vi "Tx Disable channel logic 1ch.vi"(6 "ready for output":bool, 9 "input valid":bool, 10 "data in":u32[](array[numeric])=[0, 0, 0, 0]) -> (0 "enable new data":bool, 1 "output valid":bool, 2 "data out":u32[](array[numeric]))   [LabVIEW 2025, in "niUSRP Stream Control (DMA) v1 FPGA.lvclass"]
uses:
  niUSRP Stream Control (DMA) v1 FPGA.lvclass
  niUSRP Stream Control (DMA) v1 FPGA.lvclass/niUSRP Stream Control (DMA) v1 FPGA.ctl
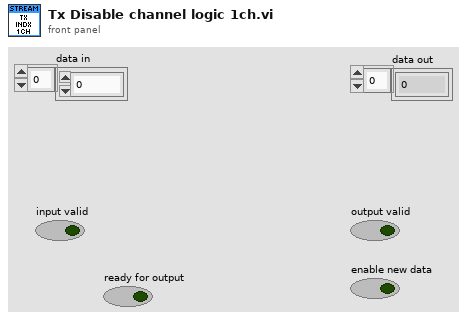
[diagram p1: front panel]
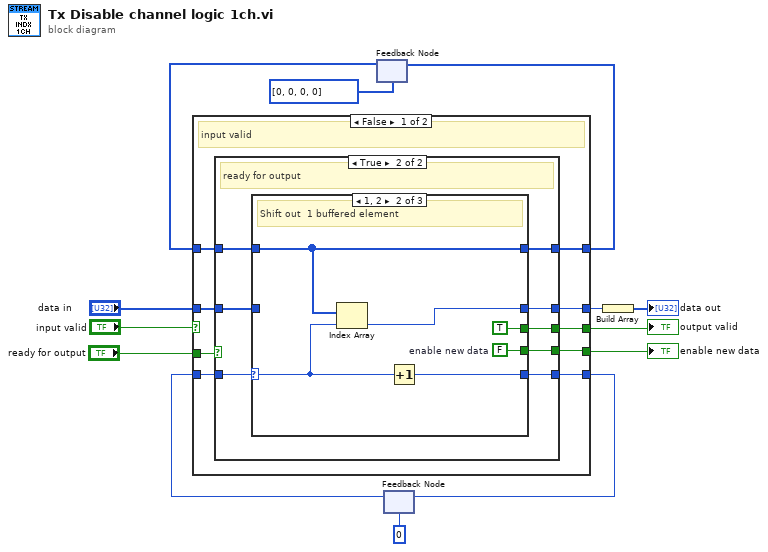
[diagram p0: block diagram]
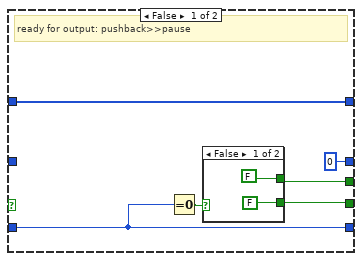
[diagram p2: hidden frame]
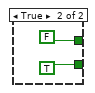
[diagram p3: hidden frame]
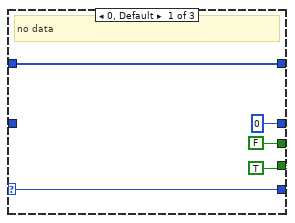
[diagram p4: hidden frame]
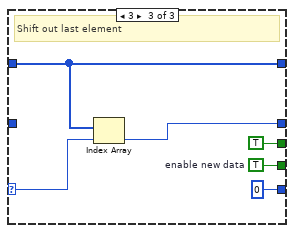
[diagram p5: hidden frame]
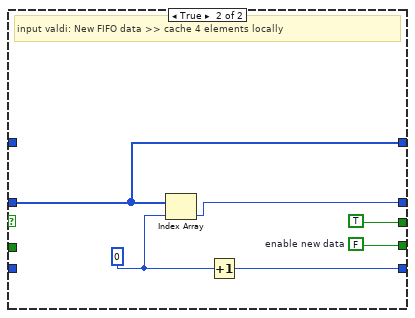
[diagram p6: hidden frame]
diagram:
  n1 = feedback #1(u32[] [0, 0, 0, 0]) -> (w12:u32[])
  n2 = feedback #2(i16 0) -> (w8:i16)
  n3 = case shown="False" "input valid" {
    tunnel: "data in" -> [w22 w59]
    tunnel: [w19 TRUE] -> w5
    tunnel: [w21 w61] -> w7
    tunnel: w8 -> [w18 _]
    tunnel: [w20 w60] -> w9
    tunnel: [w16 w59] -> w11
    tunnel: w12 -> [w17 _]
    tunnel: [w15 w58] -> w13
    tunnel: "ready for output" -> [w14 _]
    frame False {
      # "input valid"
      n4 = case shown="True" w14 {
        tunnel: w22 -> [_ w40]
        tunnel: [w27 w39] -> w21
        tunnel: [u32 0 w38] -> w20
        tunnel: [w26 w37] -> w19
        tunnel: w18 -> [w27 w36]
        tunnel: w17 -> [w24 w35]
        tunnel: [w24 w34] -> w16
        tunnel: [w25 w33] -> w15
        frame False {
          # "ready for output: pushback>>pause"
          n5 = Equal To 0?(x=w27) -> (x = 0?=w28:bool)
          n6 = case shown="False" w28 {
            tunnel: [FALSE TRUE] -> w25
            tunnel: [FALSE FALSE] -> w26
            frame False {
            }
            frame True {
            }
          }
        }
        frame True {
          # "ready for output"
          n7 = case shown="1, 2" w36 {
            selector: w36 -> [w44 w48 w54]
            tunnel: w40 -> [_ _ _]
            tunnel: [w44 w51 i16 0] -> w39
            tunnel: [u32 0 w50 w56] -> w38
            tunnel: [FALSE TRUE TRUE] -> w37
            tunnel: w35 -> [w41 w47 w53]
            tunnel: [w41 w47 w53] -> w34
            tunnel: [TRUE w46 w52] -> w33
            frame 0, Default {
              # "no data"
            }
            frame 1, 2 {
              w46 = FALSE  # enable new data
              # "Shift out  1 buffered element"
              n8 = Index Array(array=w47, index=w48) -> (element=w50:u32)
              n9 = Increment(x=w48) -> (x+1=w51:i16)
            }
            frame 3 {
              w52 = TRUE  # enable new data
              # "Shift out last element"
              n10 = Index Array(array=w53, index=w54) -> (element=w56:u32)
            }
          }
        }
      }
    }
    frame True {
      w58 = FALSE  # enable new data
      w62 = i16 0
      # "input valdi: New FIFO data >> cache 4 elements locally"
      n11 = Index Array(array=w59, index=w62) -> (element=w60:u32)
      n12 = Increment(x=w62) -> (x+1=w61:i16)
    }
  }
  "enable new data" <- w13
  "output valid" <- w5
  n13 = feedback-in #1(w11) -> ()
  n14 = feedback-in #2(w7) -> ()
  n15 = Build Array(w9) -> (→"data out":u32[])
